vi "Флаги форм..vi"(1 "Type":bool, 2 "C":bool, 3 "R":T2) -> (0 "FLAGS":T1)   [LabVIEW 2017]
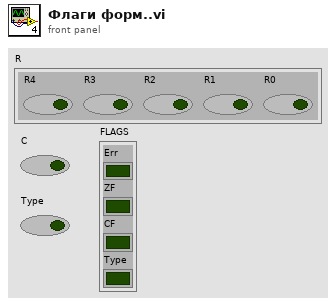
[diagram p1: front panel]
types:
  T1 = cluster{"Err":bool, "ZF":bool, "CF":bool, "Type":bool}
  T2 = cluster{"R4":bool, "R3":bool, "R2":bool, "R1":bool, "R0":bool}
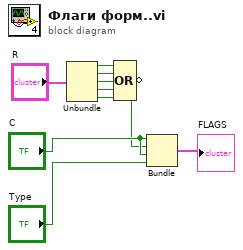
[diagram p0: block diagram]
diagram:
  n1 = Unbundle("R") -> ("R4"=w9:bool, "R3"=w8:bool, "R2"=w7:bool, "R1"=w6:bool, "R0"=w5:bool)
  n2 = Compound Arithmetic op=OR(w9, w8, w7, w6, w5) -> (invert w1:bool)
  n3 = Bundle("C"="C", w1, "C"="C", "Type"="Type") -> (→"FLAGS":cluster{"C":bool, bool, "C":bool, "Type":bool})  [unwired: 1 in]
